vi "lasersSetFrequencies_III.vi"(0 "VISA Refnum in":refnum<visa-resource-name>, 5 "f-res (Hz)":dbl, 11 "error in (no error)":errorcluster) -> (4 "405 f (Hz)":i32, 6 "532 f (Hz)":i32, 8 "662 f (Hz)":i32, 15 "error out":errorcluster)   [LabVIEW 2011]
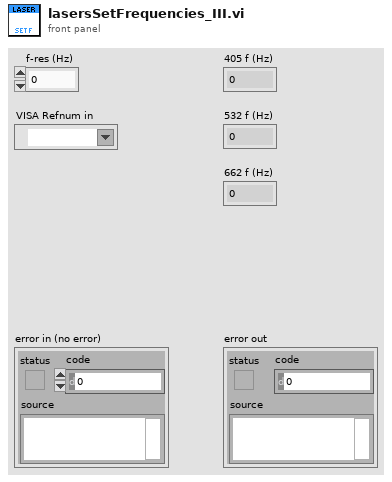
[diagram p1: front panel]
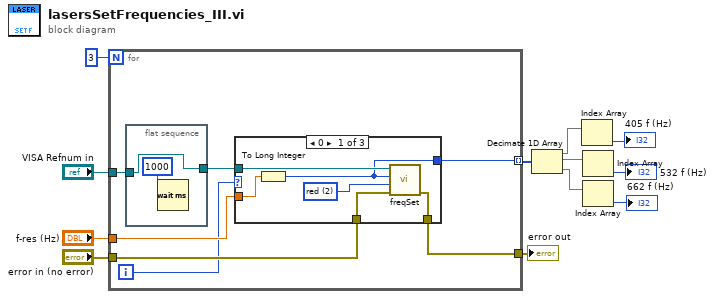
[diagram p0: block diagram]
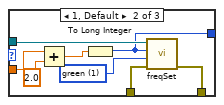
[diagram p2: hidden frame]
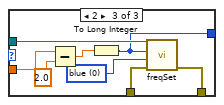
[diagram p3: hidden frame]
diagram:
  n1 = for {
    N: 3 ("Number of Lasers") -> [_]
    tunnel: [w19] -> w5
    tunnel: "error in (no error)" -> [w18]
    tunnel: "VISA Refnum in" -> [w15]
    tunnel: "f-res (Hz)" -> [w17]
    tunnel: [w13] -> w6 mode=indexing
    i -> [w16]
    n2 = flat-sequence {
      tunnel: w15 -> [w20]
      tunnel: [w20] -> w14
      frame #0 {
        n3 = Wait (ms)(milliseconds to wait=u32 1000) -> ()  [unwired: 1 out]
      }
    }
    n4 = case shown="0" w16 {
      tunnel: [w27 w35 w43] -> w19
      tunnel: w18 -> [w25 w32 w40]
      tunnel: w14 -> [w24 w31 w39]
      tunnel: w17 -> [w23 w29 w37]
      tunnel: [w22 w28 w36] -> w13
      frame 0 {
        w26 = u16 2 items=["blue", "green", "red"] ("laser")
        n5 = To Long Integer(number=w23) -> (32bit integer=w22:i32)
        n6 = call "freqSet.vi"("error in (no error)"=w25, "laser"=w26, "Freq, Hz (1370)"=w22, "Teensy Port"=w24) -> ("error out"=w27:errorcluster)  [unwired: 6 in, 1 out]
      }
      frame 1, Default {
        w34 = u16 1 items=["blue", "green", "red"] ("laser")
        n7 = Add(x=w29, y=2.0) -> (x+y=w30:dbl)
        n8 = To Long Integer(number=w30) -> (32bit integer=w28:i32)
        n9 = call "freqSet.vi"("error in (no error)"=w32, "laser"=w34, "Freq, Hz (1370)"=w28, "Teensy Port"=w31) -> ("error out"=w35:errorcluster)  [unwired: 6 in, 1 out]
      }
      frame 2 {
        w42 = u16 0 items=["blue", "green", "red"] ("laser")
        n10 = Subtract(x=w37, y=2.0) -> (x-y=w38:dbl)
        n11 = To Long Integer(number=w38) -> (32bit integer=w36:i32)
        n12 = call "freqSet.vi"("error in (no error)"=w40, "laser"=w42, "Freq, Hz (1370)"=w36, "Teensy Port"=w39) -> ("error out"=w43:errorcluster)  [unwired: 6 in, 1 out]
      }
    }
  }
  "error out" <- w5
  n13 = Decimate 1D Array(w6) -> (w7:i32[], w9:i32[], w10:i32[])
  n14 = Index Array(array=w7) -> (element=→"405 f (Hz)":i32)  [unwired: 1 in]
  n15 = Index Array(array=w9) -> (element=→"532 f (Hz)":i32)  [unwired: 1 in]
  n16 = Index Array(array=w10) -> (element=→"662 f (Hz)":i32)  [unwired: 1 in]
